vi "GetOutputWireBranch.vi"(6 "error in":errorcluster, 9 "Terminal in":refnum<class "Terminal.lvclass">) -> (0 "error out":errorcluster, 3 "Terminal out":refnum<class "Terminal.lvclass">, 4 "branches":string, 5 "branched":bool)   [LabVIEW 2014, in "Raspberry Pi Compatible Compiler for LabVIEW.lvlib" / "Terminal.lvclass"]
uses:
  Terminal.lvclass
  Python/Parsing/ListTypesTD.ctl
  Python/Parsing/Python Functions.lvlib
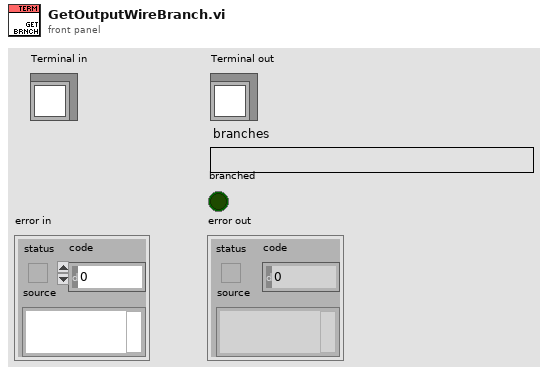
[diagram p1: front panel]
types:
  T1 = typedef "Raspberry Pi Compatible Compiler for LabVIEW.lvlib/Python Functions.lvlib/ListTypesTD.ctl" = enum16{"list", "tuple", "parameter list", "output list", "return values"}
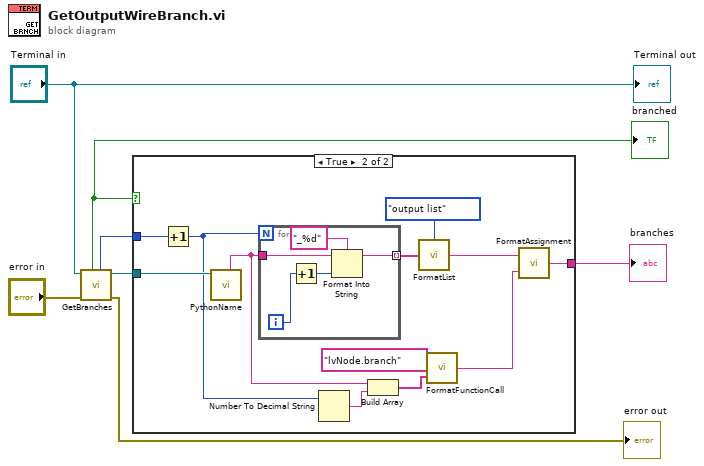
[diagram p0: block diagram]
diagram:
  n1 = call "GetBranches.vi"("error in"="error in", "Terminal in"="Terminal in") -> ("error out"=→"error out":errorcluster, "Terminal out"=w7:refnum<class "Terminal.lvclass">, "branches"=w6:i32, "wire branched"=w1:bool)  [unwired: 4 in]
  "branched" <- w1
  n2 = case shown="True" w1 {
    tunnel: w7 -> [_ w19]
    tunnel: w6 -> [_ w11]
    tunnel: [_ w9] -> w2
    frame False {
    }
    frame True {
      n3 = Increment(x=w11) -> (x+1=w8:i32)
      n4 = call-dynamic "PythonName.vi"("Terminal in"=w19) -> ("name"=w13:string)  [unwired: 7 in, 3 out]
      n5 = for {
        N: w8 -> [_]
        tunnel: w13 -> [w24]
        tunnel: [w21] -> w18 mode=indexing
        i -> [w23]
        n6 = Increment(x=w23) -> (x+1=w22:i32)
        n7 = Format Into String(format string="_%d", initial string=w24, w22) -> (resulting string=w21:string)  [unwired: 1 in, 1 out]
      }
      n8 = Number To Decimal String(number=w8) -> (decimal integer string=w12:string)  [unwired: 1 in]
      n9 = Build Array(w13, w12) -> (w10:string[])
      n10 = call "FormatList.vi"("values"=w18, "type"=ListTypesTD."output list") -> ("python object"=w16:string)
      n11 = call "FormatFunctionCall.vi"("parameters"=w10, "function"="lvNode.branch") -> ("python object"=w15:string)
      n12 = call "FormatAssignment.vi"("value"=w15, "name"=w16) -> ("python assignment"=w9:string)
    }
  }
  "branches" <- w2
  "Terminal out" <- "Terminal in"
